vi "Save CCD thermal background.vi"(0 "Data Spectrum":dbl[](array[numeric]), 2 "Save: CCD Thermal Background":bool) -> (6 "Status":string)   [LabVIEW 2009]
uses:
  <vilib>/Utility/file.llb/Write To Spreadsheet File (DBL).vi
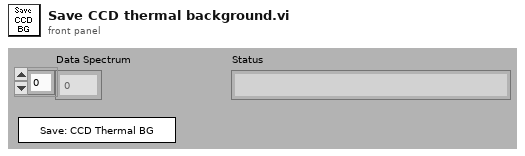
[diagram p1: front panel]
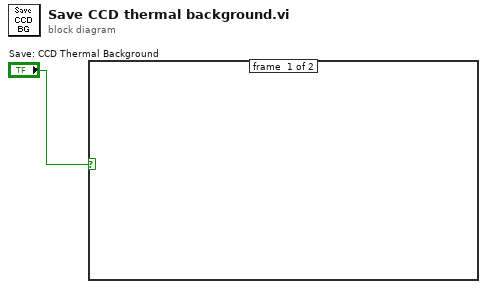
[diagram p0: block diagram]
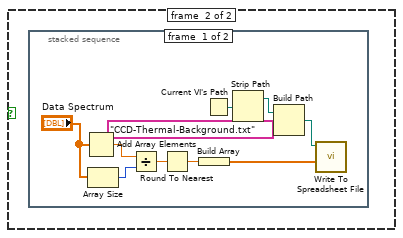
[diagram p2: hidden frame]
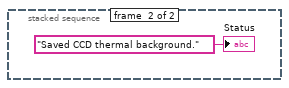
[diagram p3: hidden frame]
diagram:
  n1 = case shown="True" "Save: CCD Thermal Background" {
    frame #0 {
    }
    frame #1 {
      n2 = stacked-sequence {
        frame #0 {
          n3 = Add Array Elements(numeric array="Data Spectrum") -> (sum=w9:dbl)
          n4 = Array Size(array="Data Spectrum") -> (size(s)=w10:i32)
          n5 = Divide(x=w9, y=w10) -> (x/y=w11:dbl)
          n6 = Round To Nearest(number=w11) -> (nearest integer value=w8:dbl)
          n7 = Build Array(w8) -> (w3:dbl[])
          n8 = Current VI's Path() -> (path=w6:path)
          n9 = Strip Path(path=w6) -> (stripped path=w7:path)  [unwired: 1 out]
          n10 = Build Path(base path=w7, name or relative path="CCD-Thermal-Background.txt") -> (appended path=w4:path)
          n11 = call-poly <vilib>:"Write To Spreadsheet File.vi"("1D data"=w3, "file path (dialog if empty)"=w4) -> ()  [unwired: 6 in, 1 out]
        }
        frame #1 {
          "Status" <- "Saved CCD thermal background." ("Status")
        }
      }
    }
  }
